vi "SENS_OFFS_CW.vi"(0 "VISA IN":refnum<visa-resource-name>, 1 "CW Overide ON/OFF":bool, 5 "error in":errorcluster, 7 "Channel":i32) -> (14 "VISA Out":refnum<visa-resource-name>, 19 "error out":errorcluster)   [LabVIEW 2018, in "PNA-X.lvlib"]
doc: "SENSe<cnum>:OFFSet:CW <bool> \n(Read-Write) Turns stimulus CW Override mode ON or OFF. Use this setting to establish a fixed \n(CW) stimulus frequency while measuring the Response over a swept frequency range. \nParameters \n<cnum> Any existing channel number. If unspecified, value is set to 1 \n<bool> ON (or 1) - turns CW override ON. \nOFF (or 0) - turns CW overide OFF. \nExamples SENS:OFFS:CW ON \nsense2:offset:cw off \nQuery Syntax SENSe<cnum>:OFFSet:CW? \nReturn Type Boolean \nDefault OFF"
uses:
  PNA-X.lvlib
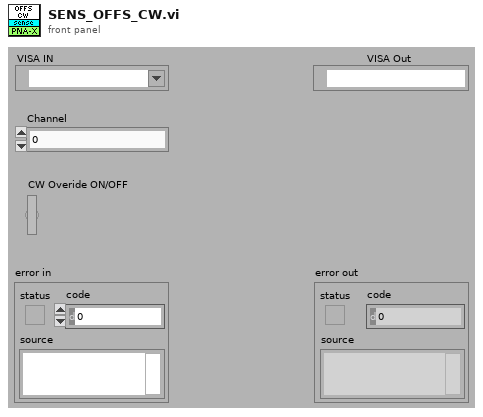
[diagram p1: front panel]
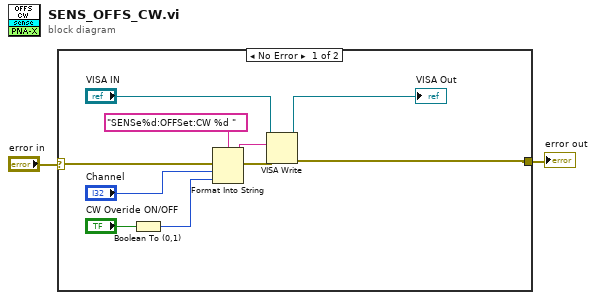
[diagram p0: block diagram]
diagram:
  n1 = case shown="No Error" "error in" {
    selector: "error in" -> [w12 w13]
    tunnel: [w7 w13] -> w1
    frame No Error {
      n2 = Boolean To (0,1)(Boolean="CW Overide ON/OFF") -> (0, 1=w3:i16)
      n3 = Format Into String(format string="SENSe%d:OFFSet:CW %d " ("Cmdline"), error in=w12, "Channel", w3) -> (resulting string=w10:string, error out=w11:errorcluster)  [unwired: 1 in]
      n4 = VISA Write(VISA resource name="VISA IN", write buffer=w10, error in (no error)=w11) -> (VISA resource name out=→"VISA Out":refnum<visa-resource-name>, error out=w7:errorcluster)  [unwired: 1 out]
    }
    frame Error {
    }
  }
  "error out" <- w1
